vi "getLevel.vi"(6 "Output Channel":T1, 8 "error in (no error)":errorcluster, 11 "Inst.RP100 in":refnum<class "Inst.RP100.lvclass">) -> (0 "error out":errorcluster, 2 "Level (V)":dbl, 3 "Inst.RP100 out":refnum<class "Inst.RP100.lvclass">)   [LabVIEW 2019, in "Inst.RP100.lvclass"]
uses:
  Inst.RP100.lvclass
  Typedefs/Channel--Num.ctl
  Typedefs/Inst.RP100.Commands--Enum.ctl
  Typedefs/getLevel--Cluster.ctl
  76e71197-b2f6-4e88-bdc7-a729cadb6927.vi
  76e71197-b2f6-4e88-bdc7-a729cadb6927.vi/775ac37a-5773-478b-a3be-b4793688c2d6.vi
  76e71197-b2f6-4e88-bdc7-a729cadb6927.vi/775ac37a-5773-478b-a3be-b4793688c2d6.vi/42ff71f4-ea9c-4d10-ac80-c5192fc06616.vi
  76e71197-b2f6-4e88-bdc7-a729cadb6927.vi/775ac37a-5773-478b-a3be-b4793688c2d6.vi/f9471b95-73a3-4ebd-ae25-3cba6cc34396.vi
  <vilib>/Utility/Data Type/Get Type Information.vi
  <vilib>/JDP Science/JSONtext/JSON text to Variant.vi
  <vilib>/JDP Science/JSONtext/LVClass Serializer/JSONtext LVClass Serializer.lvclass
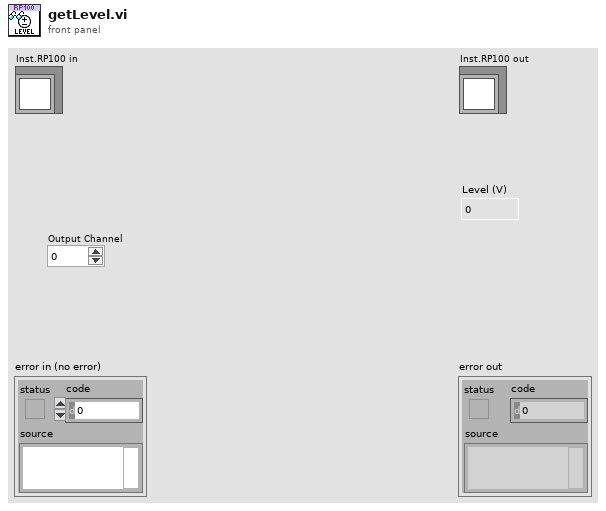
[diagram p1: front panel]
types:
  T1 = typedef "Inst.RP100.lvclass/Channel--Num.ctl" = i32
  T2 = typedef "Inst.RP100.lvclass/getLevel--Cluster.ctl" = cluster{"Channel":T1}
  T3 = typedef "Inst.RP100.lvclass/Inst.RP100.Commands--Enum.ctl" = enum16{"setState", "setLevel", "getLevel"}
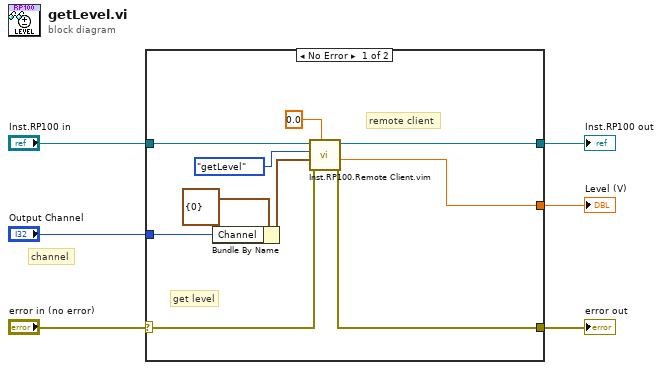
[diagram p0: block diagram]
diagram:
  # "channel"
  n1 = case shown="No Error" "error in (no error)" {
    selector: "error in (no error)" -> [w7 w18]
    tunnel: [w11 w18] -> w5
    tunnel: "Inst.RP100 in" -> [w16 w17]
    tunnel: [w15 w17] -> w3
    tunnel: [w12 _] -> w1
    tunnel: "Output Channel" -> [w9 _]
    frame No Error {
      # "remote client"
      # "get level"
      n2 = Bundle By Name(cluster=T2 {"Channel"=0} ("getLevel"), "Channel"=w9) -> (w8:T2)
      n3 = call "Inst.RP100.Remote Client.vim"("Data Out type"=0.0, "error in (no error)"=w7, "params"=w8, "Commands"=Inst.RP100.Commands--Enum."getLevel", "Inst.RP100 in"=w16) -> ("error out"=w11:errorcluster, "Data out"=w12:dbl, "Inst.RP100 out"=w15:refnum<class "Inst.RP100.lvclass">)  [unwired: 4 in]
    }
    frame Error {
    }
  }
  "error out" <- w5
  "Inst.RP100 out" <- w3
  "Level (V)" <- w1
